vi "reload_data_from_default.vi"(8 "错误输入（无错误）":errorcluster, 9 "字符串":string, 10 "簇":T25, 11 "配置":T1 {"串口通信UI"."Format" items=["标准帧", "扩展帧"]; "串口通信UI"."Type" items=["数据帧", "远程帧"]; "串口通信UI"."ID" format="0x%x"; "串口通信UI"."Fliter" items=["接收所有类型"=1, "只接收标准帧"=2, "只接收扩展帧"=3]; "串口通信UI"."kBaudRate" items=["5k bps"=1, "10k bps"=2, "20k bps"=3, "40k bps"=4, "50k bps"=5, "80k bps"=6, "100k bps"=7, "125k bps"=8, "200k bps"=9, "250k bps"=10, "400k bps"=11, "500k bps"=12, "666k bps"=13, "800k bps"=14, "1000k bps"=15, "33.33k bps"=16, "66.66k bps"=17, "83.33k bps"=18]; "串口通信UI"."Mode" items=["正常工作", "仅侦听模式", "自测模式（环回）"]; "串口通信UI"."InitFlag" items=["使用界面设置参数"=1]; "串口通信UI"."AccMask" format="%08x"; "串口通信UI"."AccCode" format="%08x"; "串口通信UI"."Channel" items=["通道1", "通道2"]; "串口通信UI"."DevType" items=["USB-CAN"=3, "USB-CAN2"=4]; "安全报警UI"."操作 8" items=["产生报警信息（不发声），等待手动操作", "产生报警信息（发声），等待手动操作", "产生报警信息（不发声），自动刹车", "产生报警信息（发声），自动刹车", "产生报警信息（不发声），立即自动断电，开启泄放电阻", "产生报警信息（发声），立即自动断电，开启泄放电阻"]; "安全报警UI"."操作 7" items=["产生报警信息（不发声），等待手动操作", "产生报警信息（发声），等待手动操作", "产生报警信息（不发声），自动刹车", "产生报警信息（发声），自动刹车", "产生报警信息（不发声），立即自动断电，开启泄放电阻", "产生报警信息（发声），立即自动断电，开启泄放电阻"]; "安全报警UI"."操作 6" items=["产生报警信息（不发声），等待手动操作", "产生报警信息（发声），等待手动操作", "产生报警信息（不发声），自动刹车", "产生报警信息（发声），自动刹车", "产生报警信息（不发声），立即自动断电，开启泄放电阻", "产生报警信息（发声），立即自动断电，开启泄放电阻"]; "安全报警UI"."操作 5" items=["产生报警信息（不发声），等待手动操作", "产生报警信息（发声），等待手动操作", "产生报警信息（不发声），自动刹车", "产生报警信息（发声），自动刹车", "产生报警信息（不发声），立即自动断电，开启泄放电阻", "产生报警信息（发声），立即自动断电，开启泄放电阻"]; "安全报警UI"."操作 4" items=["产生报警信息（不发声），等待手动操作", "产生报警信息（发声），等待手动操作", "产生报警信息（不发声），自动刹车", "产生报警信息（发声），自动刹车", "产生报警信息（不发声），立即自动断电，开启泄放电阻", "产生报警信息（发声），立即自动断电，开启泄放电阻"]; "安全报警UI"."操作 3" items=["产生报警信息（不发声），等待手动操作", "产生报警信息（发声），等待手动操作", "产生报警信息（不发声），自动刹车", "产生报警信息（发声），自动刹车", "产生报警信息（不发声），立即自动断电，开启泄放电阻", "产生报警信息（发声），立即自动断电，开启泄放电阻"]; "安全报警UI"."操作 2" items=["产生报警信息（不发声），等待手动操作", "产生报警信息（发声），等待手动操作", "产生报警信息（不发声），自动刹车", "产生报警信息（发声），自动刹车", "产生报警信息（不发声），立即自动断电，开启泄放电阻", "产生报警信息（发声），立即自动断电，开启泄放电阻"]; "安全报警UI"."操作" items=["产生报警信息（不发声），等待手动操作", "产生报警信息（发声），等待手动操作", "产生报警信息（不发声），自动刹车", "产生报警信息（发声），自动刹车", "产生报警信息（不发声），立即自动断电，开启泄放电阻", "产生报警信息（发声），立即自动断电，开启泄放电阻"]; "串口通信配置"."DevType" items=["USB-CAN"=3, "USB-CAN2"=4]; "串口通信配置"."CanIndex" items=["通道1", "通道2"]; "串口通信配置"."VCI_INIT_CONFIG"."Fliter" items=["接收所有类型"=3, "只接收标准帧"=4, "只接收扩展帧"=7]; "串口通信配置"."VCI_INIT_CONFIG"."Mode" items=["正常工作", "自测模式（环回）", "仅侦听模式"]; "串口通信配置"."VCI_INIT_CONFIG"."InitFlag" items=["使用Flash参数", "使用界面设置参数"]}) -> (0 "错误输出":errorcluster, 3 "配置输出":T1 {"串口通信UI"."Format" items=["标准帧", "扩展帧"]; "串口通信UI"."Type" items=["数据帧", "远程帧"]; "串口通信UI"."ID" format="0x%x"; "串口通信UI"."Fliter" items=["接收所有类型"=1, "只接收标准帧"=2, "只接收扩展帧"=3]; "串口通信UI"."kBaudRate" items=["5k bps"=1, "10k bps"=2, "20k bps"=3, "40k bps"=4, "50k bps"=5, "80k bps"=6, "100k bps"=7, "125k bps"=8, "200k bps"=9, "250k bps"=10, "400k bps"=11, "500k bps"=12, "666k bps"=13, "800k bps"=14, "1000k bps"=15, "33.33k bps"=16, "66.66k bps"=17, "83.33k bps"=18]; "串口通信UI"."Mode" items=["正常工作", "仅侦听模式", "自测模式（环回）"]; "串口通信UI"."InitFlag" items=["使用界面设置参数"=1]; "串口通信UI"."AccMask" format="%08x"; "串口通信UI"."AccCode" format="%08x"; "串口通信UI"."Channel" items=["通道1", "通道2"]; "串口通信UI"."DevType" items=["USB-CAN"=3, "USB-CAN2"=4]; "安全报警UI"."操作 8" items=["产生报警信息（不发声），等待手动操作", "产生报警信息（发声），等待手动操作", "产生报警信息（不发声），自动刹车", "产生报警信息（发声），自动刹车", "产生报警信息（不发声），立即自动断电，开启泄放电阻", "产生报警信息（发声），立即自动断电，开启泄放电阻"]; "安全报警UI"."操作 7" items=["产生报警信息（不发声），等待手动操作", "产生报警信息（发声），等待手动操作", "产生报警信息（不发声），自动刹车", "产生报警信息（发声），自动刹车", "产生报警信息（不发声），立即自动断电，开启泄放电阻", "产生报警信息（发声），立即自动断电，开启泄放电阻"]; "安全报警UI"."操作 6" items=["产生报警信息（不发声），等待手动操作", "产生报警信息（发声），等待手动操作", "产生报警信息（不发声），自动刹车", "产生报警信息（发声），自动刹车", "产生报警信息（不发声），立即自动断电，开启泄放电阻", "产生报警信息（发声），立即自动断电，开启泄放电阻"]; "安全报警UI"."操作 5" items=["产生报警信息（不发声），等待手动操作", "产生报警信息（发声），等待手动操作", "产生报警信息（不发声），自动刹车", "产生报警信息（发声），自动刹车", "产生报警信息（不发声），立即自动断电，开启泄放电阻", "产生报警信息（发声），立即自动断电，开启泄放电阻"]; "安全报警UI"."操作 4" items=["产生报警信息（不发声），等待手动操作", "产生报警信息（发声），等待手动操作", "产生报警信息（不发声），自动刹车", "产生报警信息（发声），自动刹车", "产生报警信息（不发声），立即自动断电，开启泄放电阻", "产生报警信息（发声），立即自动断电，开启泄放电阻"]; "安全报警UI"."操作 3" items=["产生报警信息（不发声），等待手动操作", "产生报警信息（发声），等待手动操作", "产生报警信息（不发声），自动刹车", "产生报警信息（发声），自动刹车", "产生报警信息（不发声），立即自动断电，开启泄放电阻", "产生报警信息（发声），立即自动断电，开启泄放电阻"]; "安全报警UI"."操作 2" items=["产生报警信息（不发声），等待手动操作", "产生报警信息（发声），等待手动操作", "产生报警信息（不发声），自动刹车", "产生报警信息（发声），自动刹车", "产生报警信息（不发声），立即自动断电，开启泄放电阻", "产生报警信息（发声），立即自动断电，开启泄放电阻"]; "安全报警UI"."操作" items=["产生报警信息（不发声），等待手动操作", "产生报警信息（发声），等待手动操作", "产生报警信息（不发声），自动刹车", "产生报警信息（发声），自动刹车", "产生报警信息（不发声），立即自动断电，开启泄放电阻", "产生报警信息（发声），立即自动断电，开启泄放电阻"]; "串口通信配置"."DevType" items=["USB-CAN"=3, "USB-CAN2"=4]; "串口通信配置"."CanIndex" items=["通道1", "通道2"]; "串口通信配置"."VCI_INIT_CONFIG"."Fliter" items=["接收所有类型"=3, "只接收标准帧"=4, "只接收扩展帧"=7]; "串口通信配置"."VCI_INIT_CONFIG"."Mode" items=["正常工作", "自测模式（环回）", "仅侦听模式"]; "串口通信配置"."VCI_INIT_CONFIG"."InitFlag" items=["使用Flash参数", "使用界面设置参数"]})   [LabVIEW 2018, in "UI.lvlib"]
uses:
  UI.lvlib
  Settings/Settings.ctl
  Acquisition/Hardware Configuration.ctl
  Acquisition/Signal Type.ctl
  canstatus.ctl
  <vilib>/Utility/xml.llb/Read From XML File(string).vi
  Settings/Settings.lvlib
  Acquisition/Acquisition.lvlib
panel:
  # "参数配置文件"
  # "输入数据文件"
  # "EHA电机"
  # "模拟电机"
  # "注：每次运行实验时销毁现有所有图像"
  # "参数配置文件"
  # "输入数据文件"
  # "EHA电机"
  # "模拟电机"
  # "注：每次运行实验时销毁现有所有图像"
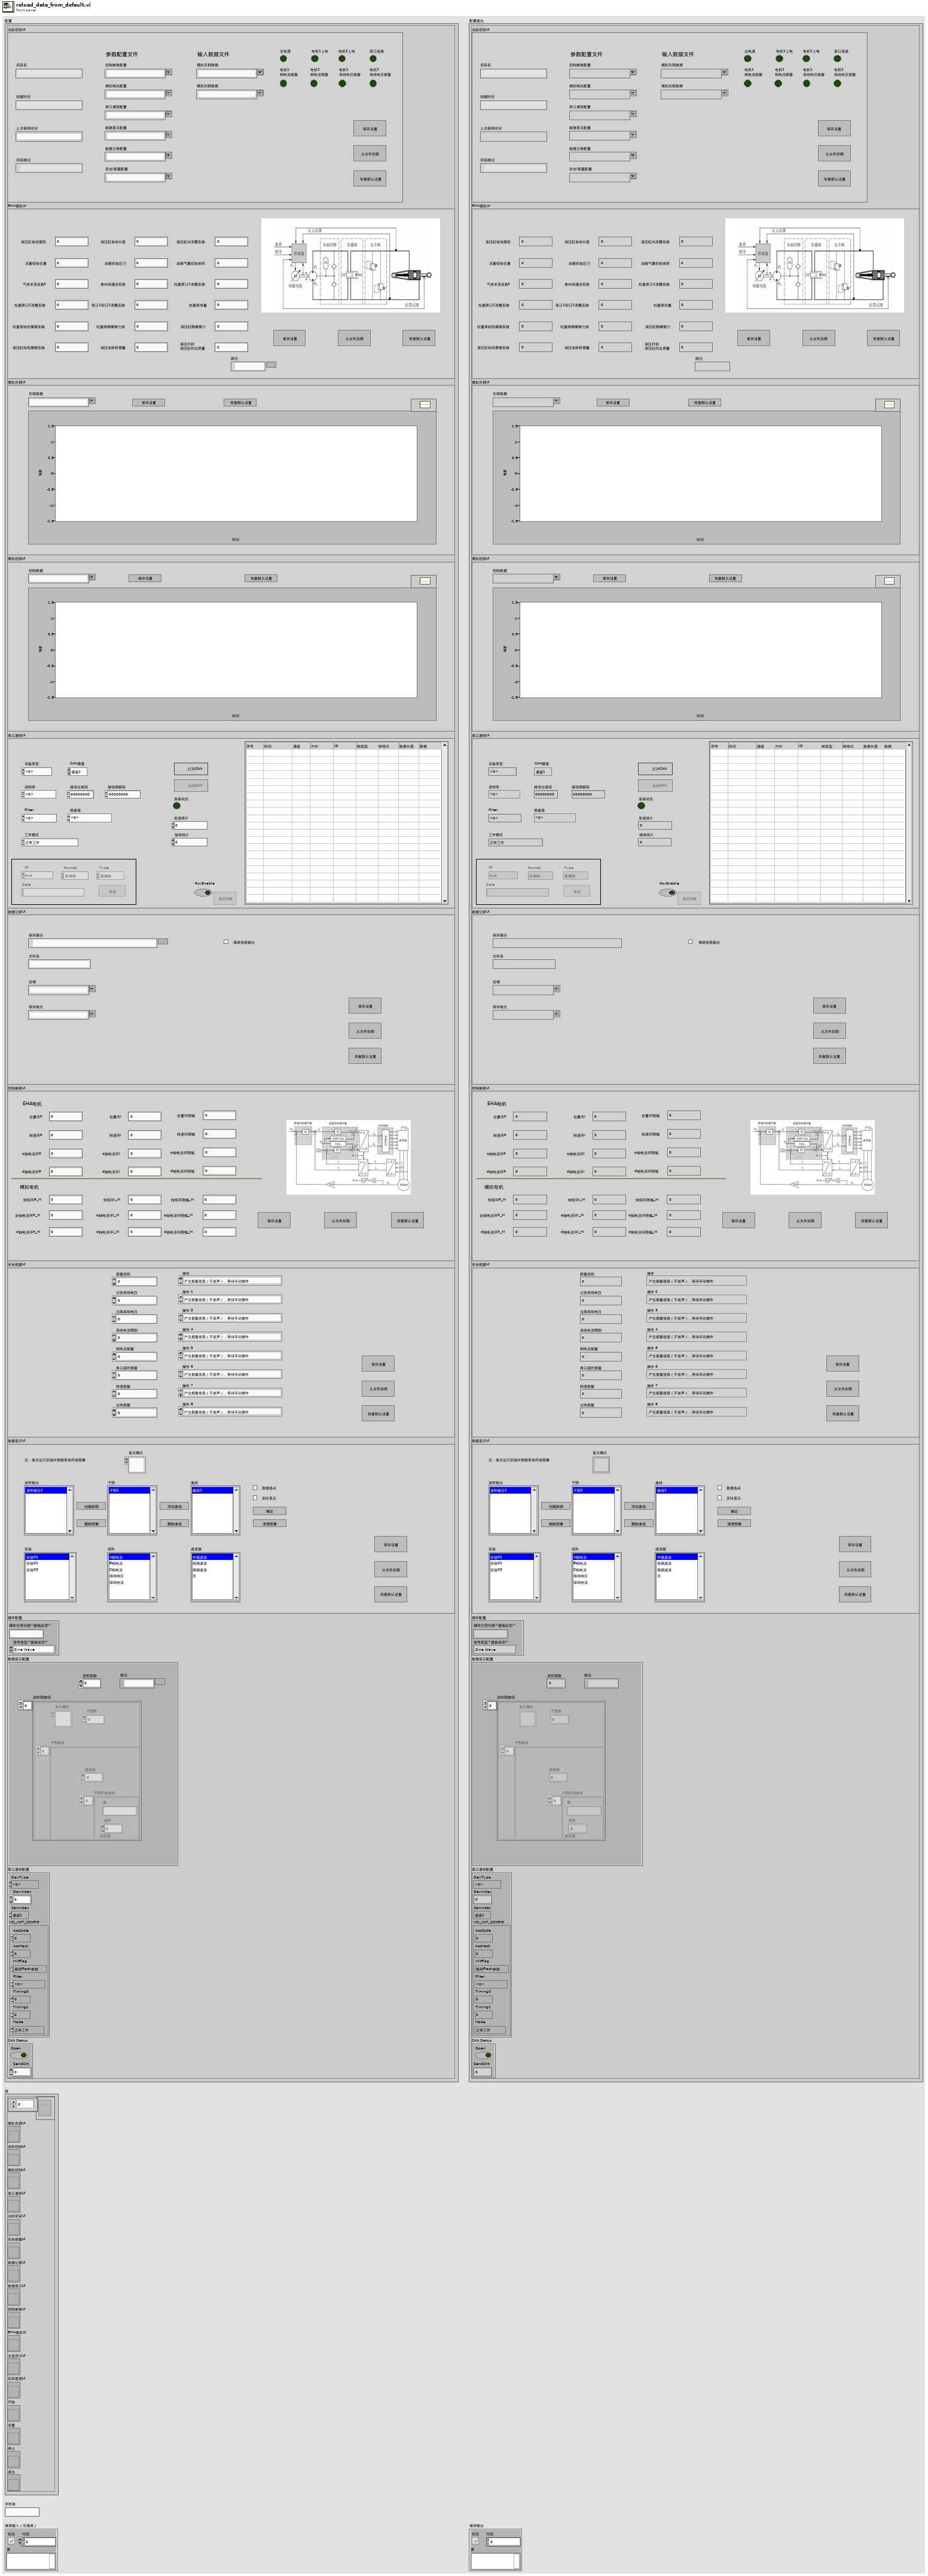
[diagram p1: front panel]
types:
  T1 = typedef "Settings.lvlib/Settings.ctl" = cluster{"当前项目UI":T2, "EHA模拟UI":T3, "模拟负载UI":T4, "模拟控制UI":T5, "串口通信UI":T6, "数据记录UI":T12, "控制参数UI":T13, "安全报警UI":T14, "数据显示UI":T15, "硬件配置":T16, "数据显示配置":T18, "串口通信配置":T22, "CAN Status":T24}
  T2 = typedef "控件 5.ctl" = cluster{"控制参数配置":string, "模拟响应配置":string, "串口通信配置":string, "数据显示配置":string, "数据记录配置":string, "安全/报警配置":string, "模拟负载数据":string, "模拟加载数据":string, "总电源":bool, "电机1上电":bool, "电机2上电":bool, "串口连接":bool, "电机1\n相电流报警":bool, "电机2\n相电流报警":bool, "电机1\n母线电压报警":bool, "电机2\n母线电压报警":bool, "保存设置":bool, "从文件加载":bool, "恢复默认设置":bool, "路径":path, "项目路径":path, "项目名":string, "创建时间":string, "上次使用时间":string}
  T3 = typedef "EHA模拟UI.ctl" = cluster{"液压缸有效面积":dbl, "活塞初始位置":dbl, "气体多变系数k":dbl, "柱塞泵口2泄露系数":dbl, "柱塞泵粘性摩擦系数":dbl, "液压缸粘性摩擦系数":dbl, "液压缸有效长度":dbl, "油箱初始压力":dbl, "单向阀通流系数":dbl, "泵口1到口2泄露系数":dbl, "柱塞泵静摩擦力矩":dbl, "液压油体积模量":dbl, "保存设置":bool, "从文件加载":bool, "恢复默认设置":bool, "路径":path, "液压缸内泄露系数":dbl, "油箱气囊初始体积":dbl, "柱塞泵口1泄露系数":dbl, "柱塞泵排量":dbl, "液压缸静摩擦力":dbl, "液压杆到\n液压缸的总质量":dbl}
  T4 = typedef "控件 9.ctl" = cluster{"负载数据":string, "负载数据 2":waveform(dbl)[], "保存设置":bool, "恢复默认设置":bool}
  T5 = typedef "控件 7.ctl" = cluster{"控制数据":string, "负载数据 2":waveform(dbl)[], "保存设置":bool, "恢复默认设置":bool}
  T6 = typedef "控件 6.ctl" = cluster{"DevType":T7, "Channel":T8, "AccCode":u32, "AccMask":u32, "InitFlag":T9, "Mode":T10, "kBaudRate":u8, "Fliter":T11, "Open":bool, "Close":bool, "连接状态":bool, "SendCnt":u32, "RecvCnt":u32, "Send":bool, "ID":u32, "Data":string, "Type":u8, "Format":u8, "Clear":bool, "list":i32, "路径":path, "RcvEnable":bool}
  T7 = typedef "can库.lvlib/ControlCAN.lvlib/DevType.ctl" = u32
  T8 = typedef "can库.lvlib/ControlCAN.lvlib/CAN Channel.ctl" = u32
  T9 = typedef "can库.lvlib/ControlCAN.lvlib/InitFlag.ctl" = u32
  T10 = typedef "can库.lvlib/ControlCAN.lvlib/Mode.ctl" = u8
  T11 = typedef "can库.lvlib/ControlCAN.lvlib/Fliter.ctl" = u8
  T12 = typedef "控件 3.ctl" = cluster{"保存路径":path, "文件名":string, "后缀":string, "保存格式":string, "复选框":bool, "保存设置":bool, "从文件加载":bool, "恢复默认设置":bool, "路径":path, "TDMS文件引用":refnum<k34>}
  T13 = typedef "控件 1.ctl" = cluster{"d轴电流环P_M":dbl, "转速环P":dbl, "q轴电流环P":dbl, "d轴电流环P":dbl, "转矩环P_M":dbl, "去轴电流环P_M":dbl, "转速环I":dbl, "q轴电流环I":dbl, "d轴电流环I":dbl, "转矩环I_M":dbl, "q轴电流环I_M":dbl, "d轴电流环I_M":dbl, "保存设置":bool, "从文件加载":bool, "恢复默认设置":bool, "路径":path, "位置环P":dbl, "位置环I":dbl, "转速环限幅":dbl, "q轴电流环限幅":dbl, "d轴电流环限幅":dbl, "位置环限幅":dbl, "转矩环限幅_M":dbl, "q轴电流环限幅_M":dbl, "d轴电流环限幅_M":dbl}
  T14 = typedef "控件 4.ctl" = cluster{"报警扭矩":dbl, "过低母线电压":dbl, "过高母线电压":dbl, "母线电流限制":dbl, "相电流报警":dbl, "串口超时报警":dbl, "转速报警":dbl, "过热报警":dbl, "操作":u16, "操作 2":u16, "操作 3":u16, "操作 4":u16, "操作 5":u16, "操作 6":u16, "操作 7":u16, "操作 8":u16, "保存设置":bool, "从文件加载":bool, "恢复默认设置":bool, "路径":path}
  T15 = typedef "控件 2.ctl" = cluster{"保存设置":bool, "从文件加载":bool, "恢复默认设置":bool, "实验":i32, "波形输出":i32, "组件":i32, "曲线":i32, "滤波器":i32, "删除曲线":bool, "清理图像":bool, "添加曲线":bool, "数据选点":bool, "确定按钮":bool, "实时显示":bool, "子图":i32, "显示模式":u16, "路径":path, "删除图像":bool, "创建新图":bool}
  T16 = typedef "Acquisition.lvlib/Hardware Configuration.ctl" = cluster{"硬件引用句柄<替换此项>":string, "信号类型<替换该项>":T17}
  T17 = typedef "Acquisition.lvlib/Signal Type.ctl" = enum16{"Sine Wave", "Square with Noise"}
  T18 = typedef "波形图簇.ctl" = cluster{"波形图数":u32, "波形图数组":T19[], "路径":path}
  T19 = typedef "波形图.ctl" = cluster{"显示模式":u16, "子图数":u32, "子图数组":T20[]}
  T20 = typedef "子图.ctl" = cluster{"子图所有曲线":T21[], "曲线数":u32}
  T21 = typedef "曲线簇.ctl" = cluster{"源":string, "组件":u32, "滤波器":u32}
  T22 = typedef "UI.lvlib/串口通信配置.ctl" = cluster{"DevType":T7, "DevIndex":u32, "CanIndex":T8, "VCI_INIT_CONFIG":T23}
  T23 = typedef "can库.lvlib/ControlCAN.lvlib/VCI_INIT_CONFIG.ctl" = cluster{"AccCode":u32, "AccMask":u32, "InitFlag":T9, "Fliter":T11, "Timing0":u8, "Timing1":u8, "Mode":T10}
  T24 = typedef "UI.lvlib/canstatus.ctl" = cluster{"Open":bool, "SendCnt":u32}
  T25 = typedef "引用簇.ctl" = cluster{"数组":refnum<vi>[], "模拟负载UI":refnum<vi>, "波形控制UI":refnum<vi>, "模拟控制UI":refnum<vi>, "串口通信UI":refnum<vi>, "当前项目UI":refnum<vi>, "安全报警UI":refnum<vi>, "数据记录UI":refnum<vi>, "数据显示UI":refnum<vi>, "控制参数UI":refnum<vi>, "EHA模拟UI":refnum<vi>, "主选项卡UI":refnum<vi>, "项目管理UI":refnum<vi>, "开始":refnum<vi>, "设置":refnum<vi>, "停止":refnum<vi>, "退出":refnum<vi>}
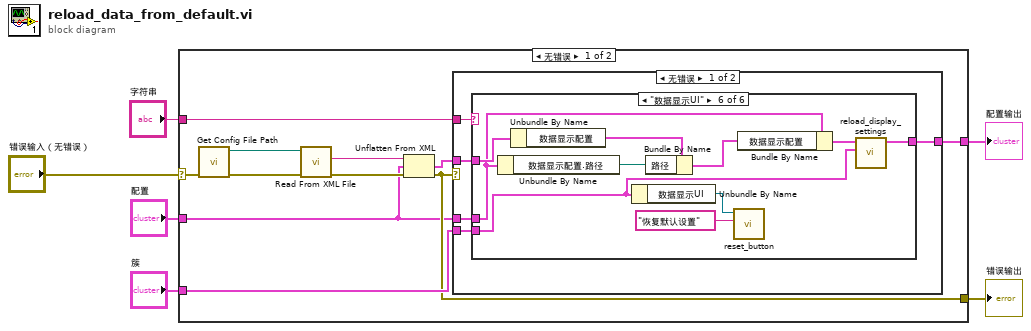
[diagram p0: block diagram]
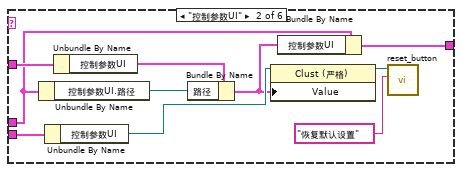
[diagram p3: hidden frame]
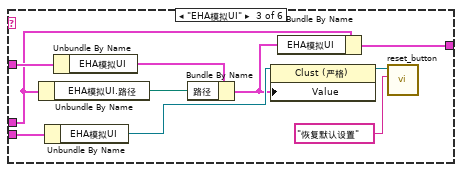
[diagram p4: hidden frame]
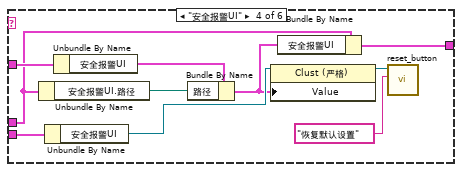
[diagram p5: hidden frame]
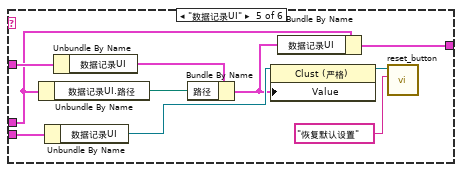
[diagram p6: hidden frame]
diagram:
  n1 = case shown="无错误" "错误输入（无错误）" {
    selector: "错误输入（无错误）" -> [w17 w76]
    tunnel: "配置" -> [w8 w75]
    tunnel: "字符串" -> [w9 _]
    tunnel: "簇" -> [w13 _]
    tunnel: [w10 w76] -> w3
    tunnel: [w7 w75] -> w1
    frame No Error {
      n2 = call "Get Config File Path.vi"("error in (no error)"=w17) -> ("error out"=w16:cluster{"状态":bool, "代码":i32, "源":string}, "XML文件路径"=w15:path)  [unwired: 9 in]
      n3 = call-poly <vilib>:"Read From XML File.vi"("error in (no error)"=w16, "XML File Path"=w15) -> ("error out"=w11:errorcluster, "XML Elements"=w14:string)  [unwired: 7 in, 1 out]
      n4 = Unflatten From XML(xml string=w14, type=w8, error in (no error)=w11) -> (value=w12:T1, error out=w10:errorcluster)
      n5 = case shown="无错误" w10 {
        tunnel: w9 -> [w22 _]
        tunnel: w13 -> [w21 _]
        tunnel: w12 -> [w20 _]
        tunnel: w8 -> [w19 w74]
        tunnel: [w18 w74] -> w7
        frame No Error {
          n6 = case shown="\"数据显示UI\"" w22 {
            tunnel: w20 -> [_ w30 w40 w50 w61 w72]
            tunnel: w21 -> [_ w32 w42 w52 w62 w66]
            tunnel: w19 -> [w23 w26 w36 w46 w56 w67]
            tunnel: [w23 w27 w37 w47 w57 w64] -> w18
            frame "假", Default {
            }
            frame "控制参数UI" {
              n7 = Unbundle By Name(w26) -> ("控制参数UI.路径"=w29:path)
              n8 = Unbundle By Name(w32) -> ("控制参数UI"=w31:refnum<vi>)
              n9 = Unbundle By Name(w30) -> ("控制参数UI"=w33:T13)
              n10 = Bundle By Name(cluster=w33, "路径"=w29) -> (w25:T13)
              n11 = property class="Clust (严格)"(reference=w31, "Value"=w25) -> (reference out=w28:refnum<vi>)  [unwired: 1 in, 1 out]
              n12 = Bundle By Name(cluster=w26, "控制参数UI"=w25) -> (w27:T1)
              n13 = call "reset_button.vi"("字符串"="恢复默认设置", "Cluster输入"=w28) -> ()  [unwired: 9 in, 1 out]
            }
            frame "EHA模拟UI" {
              n14 = Unbundle By Name(w36) -> ("EHA模拟UI.路径"=w39:path)
              n15 = Unbundle By Name(w42) -> ("EHA模拟UI"=w41:refnum<vi>)
              n16 = Unbundle By Name(w40) -> ("EHA模拟UI"=w43:T3)
              n17 = Bundle By Name(cluster=w43, "路径"=w39) -> (w35:T3)
              n18 = property class="Clust (严格)"(reference=w41, "Value"=w35) -> (reference out=w38:refnum<vi>)  [unwired: 1 in, 1 out]
              n19 = Bundle By Name(cluster=w36, "EHA模拟UI"=w35) -> (w37:T1)
              n20 = call "reset_button.vi"("字符串"="恢复默认设置", "Cluster输入"=w38) -> ()  [unwired: 9 in, 1 out]
            }
            frame "安全报警UI" {
              n21 = Unbundle By Name(w46) -> ("安全报警UI.路径"=w49:path)
              n22 = Unbundle By Name(w52) -> ("安全报警UI"=w51:refnum<vi>)
              n23 = Unbundle By Name(w50) -> ("安全报警UI"=w53:T14)
              n24 = Bundle By Name(cluster=w53, "路径"=w49) -> (w45:T14)
              n25 = property class="Clust (严格)"(reference=w51, "Value"=w45) -> (reference out=w48:refnum<vi>)  [unwired: 1 in, 1 out]
              n26 = Bundle By Name(cluster=w46, "安全报警UI"=w45) -> (w47:T1)
              n27 = call "reset_button.vi"("字符串"="恢复默认设置", "Cluster输入"=w48) -> ()  [unwired: 9 in, 1 out]
            }
            frame "数据记录UI" {
              n28 = Unbundle By Name(w56) -> ("数据记录UI.路径"=w60:path)
              n29 = Unbundle By Name(w62) -> ("数据记录UI"=w59:refnum<vi>)
              n30 = Unbundle By Name(w61) -> ("数据记录UI"=w63:T12)
              n31 = Bundle By Name(cluster=w63, "路径"=w60) -> (w55:T12)
              n32 = property class="Clust (严格)"(reference=w59, "Value"=w55) -> (reference out=w58:refnum<vi>)  [unwired: 1 in, 1 out]
              n33 = Bundle By Name(cluster=w56, "数据记录UI"=w55) -> (w57:T1)
              n34 = call "reset_button.vi"("字符串"="恢复默认设置", "Cluster输入"=w58) -> ()  [unwired: 9 in, 1 out]
            }
            frame "数据显示UI" {
              n35 = Unbundle By Name(w67) -> ("数据显示配置.路径"=w71:path)
              n36 = Unbundle By Name(w72) -> ("数据显示配置"=w73:T18)
              n37 = Unbundle By Name(w66) -> ("数据显示UI"=w69:refnum<vi>)
              n38 = Bundle By Name(cluster=w73, "路径"=w71) -> (w70:T18)
              n39 = call "reset_button.vi"("字符串"="恢复默认设置", "Cluster输入"=w69) -> ()  [unwired: 9 in, 1 out]
              n40 = Bundle By Name(cluster=w67, "数据显示配置"=w70) -> (w65:T1)
              n41 = call "reload_display_settings.vi"("簇"=w66, "配置"=w65) -> ("配置输出"=w64:T1)  [unwired: 9 in]
            }
          }
        }
        frame Error {
        }
      }
    }
    frame Error {
    }
  }
  "配置输出" <- w1
  "错误输出" <- w3
